vi "VariantToINIstring (Standard).vi"(11 "Variant-formatted Value":variant) -> (3 "String-formatted Value":string)   [LabVIEW 2013, in "OpenSerializer.lvlib" / "Serializer.PlainText.INI.lvclass"]
uses:
  Serializer.PlainText.INI.lvclass
  <vilib>/LabVIEW Open Source Project/Data Manipulation/TypeDescriptor/TypeDescriptor_GetName.vi
  <vilib>/LabVIEW Open Source Project/Data Manipulation/TypeDescriptor/TypeDescriptor_GetPString.vi
  <vilib>/LabVIEW Open Source Project/Data Manipulation/TypeDescriptor/TypeDescriptor_SetName.vi
  <vilib>/Utility/GetType.llb/Get Type Code from I16 Array And Pos.vi
  <vilib>/Utility/GetType.llb/TD_Get Array Information.vi
  <vilib>/LabVIEW Open Source Project/Data Manipulation/Conversions/Flattened nD-Array to Flattened 1D-Array.vi
  <vilib>/Utility/VariantDataType/VariantType.lvlib
  <vilib>/LabVIEW Open Source Project/Data Manipulation/Variant/OpenVariant.lvlib
  <vilib>/LabVIEW Open Source Project/Data Manipulation/TypeDescriptor/OpenDescriptor.lvlib
  Serializer.PlainText/Serializer.PlainText.lvclass
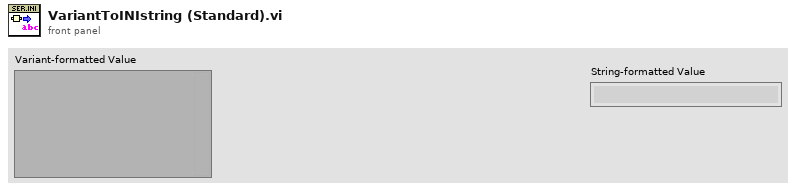
[diagram p1: front panel]
types:
  T1 = typedef "VariantType.lvlib/Type.ctl" = enum8{"Invalid Type", "Void", "I8", "I16", "I32", "I64", "U8", "U16", "U32", "U64", "Single Float", "Double Float", "Extended Float", "Single Complex", "Double Complex", "Extended Complex", "Enum U8", "Enum U16", "Enum U32", "Enum U64", "Single Float With Unit", "Double Float With Unit", "Extended Float With Unit", "Single Complex with Unit", "Double Complex with Unit", "Extended Complex with Unit", "Boolean", "String", "Path", "Picture", "Tag", "Array", "Cluster", "Variant", "LV Variant", "Waveform", "Timestamp", "Digital Waveform", "Digital Data", "ExpressData", "Refnum", "External Data", "VI", "Poly VI", "LabVIEW Class Instance", "Fixed Point"}
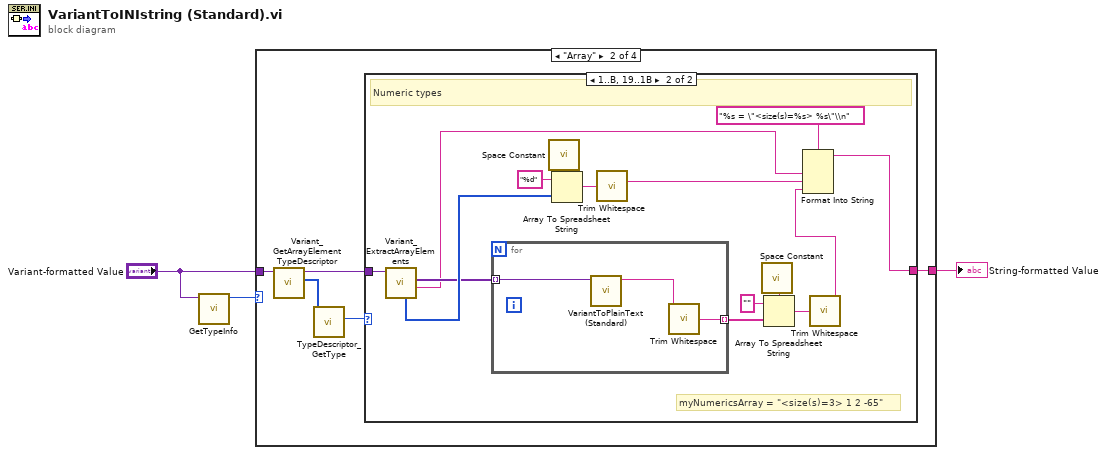
[diagram p0: block diagram]
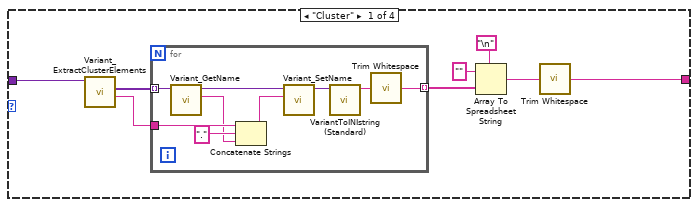
[diagram p2: hidden frame]
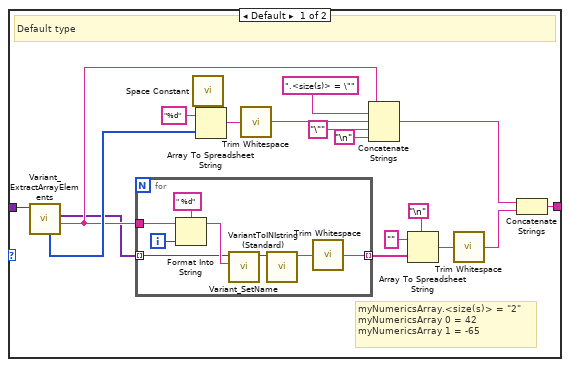
[diagram p3: hidden frame]
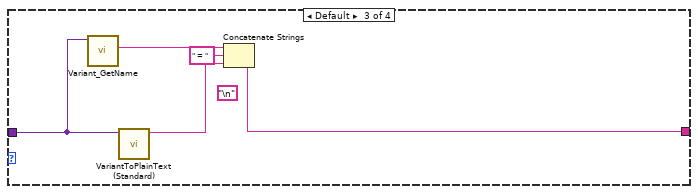
[diagram p4: hidden frame]
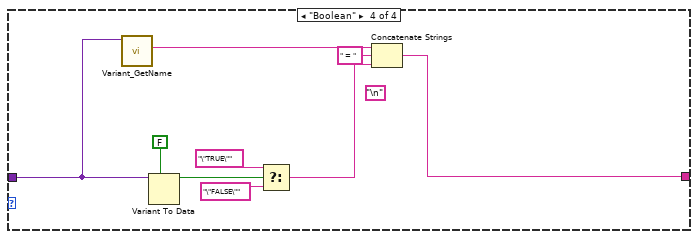
[diagram p5: hidden frame]
diagram:
  n1 = call <vilib>:"GetTypeInfo.vi"("Variant"="Variant-formatted Value") -> ("Type Enum"=w3:T1)  [unwired: 6 in, 4 out]
  n2 = case shown="\"Array\"" w3 {
    tunnel: "Variant-formatted Value" -> [w11 w23 w71 w77]
    tunnel: [w4 w25 w72 w75] -> w1
    frame "Cluster" {
      n3 = call <vilib>:"Variant_ExtractClusterElements.vi"("Cluster"=w11) -> ("name"=w7:string, "Elements"=w10:variant[])  [unwired: 8 in, 1 out]
      n4 = for {
        tunnel: w10 -> [w20] mode=indexing
        tunnel: [w12] -> w9 mode=indexing
        tunnel: w7 -> [w18]
        n5 = call <vilib>:"Variant_GetName.vi"("Variant"=w20) -> ("Name"=w17:string, "Variant dup"=w15:variant)  [unwired: 8 in, 1 out]
        n6 = Concatenate Strings(w18, "." ("string"), w17) -> (w16:string)
        n7 = call <vilib>:"Variant_SetName.vi"("Name"=w16, "Variant"=w15) -> ("Named Variant"=w14:variant)  [unwired: 9 in]
        n8 = call "VariantToINIstring (Standard).vi"("Variant-formatted Value"=w14) -> ("String-formatted Value"=w13:string)  [unwired: 10 in]
        n9 = call <vilib>:"Trim Whitespace.vi"("string"=w13) -> ("trimmed string"=w12:string)  [unwired: 1 in]
      }
      n10 = Array To Spreadsheet String(delimiter (Tab)="\n", array=w9, 3:"" ("format string")) -> (spreadsheet string=w5:string)
      n11 = call <vilib>:"Trim Whitespace.vi"("string"=w5) -> ("trimmed string"=w4:string)  [unwired: 1 in]
    }
    frame "Array" {
      n12 = call <vilib>:"Variant_GetArrayElementTypeDescriptor.vi"("Array"=w23) -> ("Element Descriptor"=w24:i16[], "Array dup"=w22:variant)  [unwired: 8 in, 1 out]
      n13 = call <vilib>:"TypeDescriptor_GetType.vi"("type descriptor"=w24) -> ("Type"=w21:u8)  [unwired: 9 in, 1 out]
      n14 = case shown="1..B, 19..1B" w21 {
        tunnel: [w43 w53] -> w25
        tunnel: w22 -> [w26 w58]
        frame Default {
          # "myNumericsArray.<size(s)> = \"2\"\nmyNumericsArray 0 = 42\nmyNumericsArray 1 = -65"
          # "Default type"
          n15 = call <vilib>:"Variant_ExtractArrayElements.vi"("Array"=w26) -> ("name"=w33:string, "Elements"=w32:variant[], "Dimensions"=w39:u32[])  [unwired: 7 in, 1 out]
          n16 = for {
            tunnel: w33 -> [w48]
            tunnel: w32 -> [w44] mode=indexing
            tunnel: [w45] -> w29 mode=indexing
            i -> [w50]
            n17 = Format Into String(format string=" %d" ("Format String"), initial string=w48, w50) -> (resulting string=w47:string)  [unwired: 1 in, 1 out]
            n18 = call <vilib>:"Variant_SetName.vi"("Name"=w47, "Variant"=w44) -> ("Named Variant"=w49:variant)  [unwired: 9 in]
            n19 = call "VariantToINIstring (Standard).vi"("Variant-formatted Value"=w49) -> ("String-formatted Value"=w46:string)  [unwired: 10 in]
            n20 = call <vilib>:"Trim Whitespace.vi"("string"=w46) -> ("trimmed string"=w45:string)  [unwired: 1 in]
          }
          n21 = call <vilib>:"Space Constant.vi"() -> ("String"=w42:string)
          n22 = Array To Spreadsheet String(delimiter (Tab)=w42, array=w39, 3:"%d" ("format string")) -> (spreadsheet string=w40:string)
          n23 = call <vilib>:"Trim Whitespace.vi"("string"=w40) -> ("trimmed string"=w35:string)  [unwired: 1 in]
          n24 = Concatenate Strings(w33, ".<size(s)> = \"" ("Substring"), w35, "\"" ("string"), "\n") -> (w34:string)
          n25 = Array To Spreadsheet String(delimiter (Tab)="\n", array=w29, 3:"" ("format string")) -> (spreadsheet string=w28:string)
          n26 = call <vilib>:"Trim Whitespace.vi"("string"=w28) -> ("trimmed string"=w27:string)  [unwired: 1 in]
          n27 = Concatenate Strings(w34, w27) -> (w43:string)
        }
        frame 1..11, 25..27 {
          # "myNumericsArray = \"<size(s)=3> 1 2 -65\""
          # "Numeric types"
          n28 = call <vilib>:"Variant_ExtractArrayElements.vi"("Array"=w58) -> ("name"=w57:string, "Elements"=w62:variant[], "Dimensions"=w63:u32[])  [unwired: 7 in, 1 out]
          n29 = for {
            tunnel: w62 -> [w68] mode=indexing
            tunnel: [w69] -> w60 mode=indexing
            n30 = call "VariantToPlainText (Standard).vi"("Variant-formatted Value"=w68) -> ("String-formatted Value"=w67:string)  [unwired: 10 in]
            n31 = call <vilib>:"Trim Whitespace.vi"("string"=w67) -> ("trimmed string"=w69:string)  [unwired: 1 in]
          }
          n32 = call <vilib>:"Space Constant.vi"() -> ("String"=w66:string)
          n33 = Array To Spreadsheet String(delimiter (Tab)=w66, array=w63, 3:"%d" ("format string")) -> (spreadsheet string=w64:string)
          n34 = call <vilib>:"Trim Whitespace.vi"("string"=w64) -> ("trimmed string"=w55:string)  [unwired: 1 in]
          n35 = call <vilib>:"Space Constant.vi"() -> ("String"=w52:string)
          n36 = Array To Spreadsheet String(delimiter (Tab)=w52, array=w60, 3:"" ("format string")) -> (spreadsheet string=w59:string)
          n37 = call <vilib>:"Trim Whitespace.vi"("string"=w59) -> ("trimmed string"=w54:string)  [unwired: 1 in]
          n38 = Format Into String(format string="%s = \"<size(s)=%s> %s\"\\n", w57, w55, w54) -> (resulting string=w53:string)  [unwired: 2 in, 1 out]
        }
      }
    }
    frame Default {
      (unwired) "\n"
      n39 = call <vilib>:"Variant_GetName.vi"("Variant"=w71) -> ("Name"=w74:string)  [unwired: 8 in, 2 out]
      n40 = call "VariantToPlainText (Standard).vi"("Variant-formatted Value"=w71) -> ("String-formatted Value"=w70:string)  [unwired: 10 in]
      n41 = Concatenate Strings(w74, " = " ("string"), w70) -> (w72:string)
    }
    frame "Boolean" {
      (unwired) "\n"
      n42 = call <vilib>:"Variant_GetName.vi"("Variant"=w77) -> ("Name"=w79:string)  [unwired: 8 in, 2 out]
      n43 = Variant To Data(type=FALSE, Variant=w77) -> (data=w82:bool)  [unwired: 1 in, 1 out]
      n44 = Select(t="\"TRUE\"", s=w82, f="\"FALSE\"") -> (s? t:f=w76:string)
      n45 = Concatenate Strings(w79, " = " ("string"), w76) -> (w75:string)
    }
  }
  "String-formatted Value" <- w1
